vi "MFC_Setpoint.vi"(8 "error in":errorcluster, 9 "index":i32, 10 "MFC Set":T1[](array[typedef])=[{"MFC Set"=[{"String"="A", "MFC set"=1000.0}, {"String"="B", "MFC set"=100.0}], "set 1"=FALSE}] {"MFC Set"."MFC set" step=10.0 format="%.2f"}, 11 "VISA Refnum in":refnum<visa-resource-name>="COM6") -> (0 "error out":errorcluster, 3 "VISA Refnum out":refnum<visa-resource-name>="COM6")   [LabVIEW 2020]
uses:
  typeDefs/MFCSet.ctl
panel:
  out "MFC Index":i32
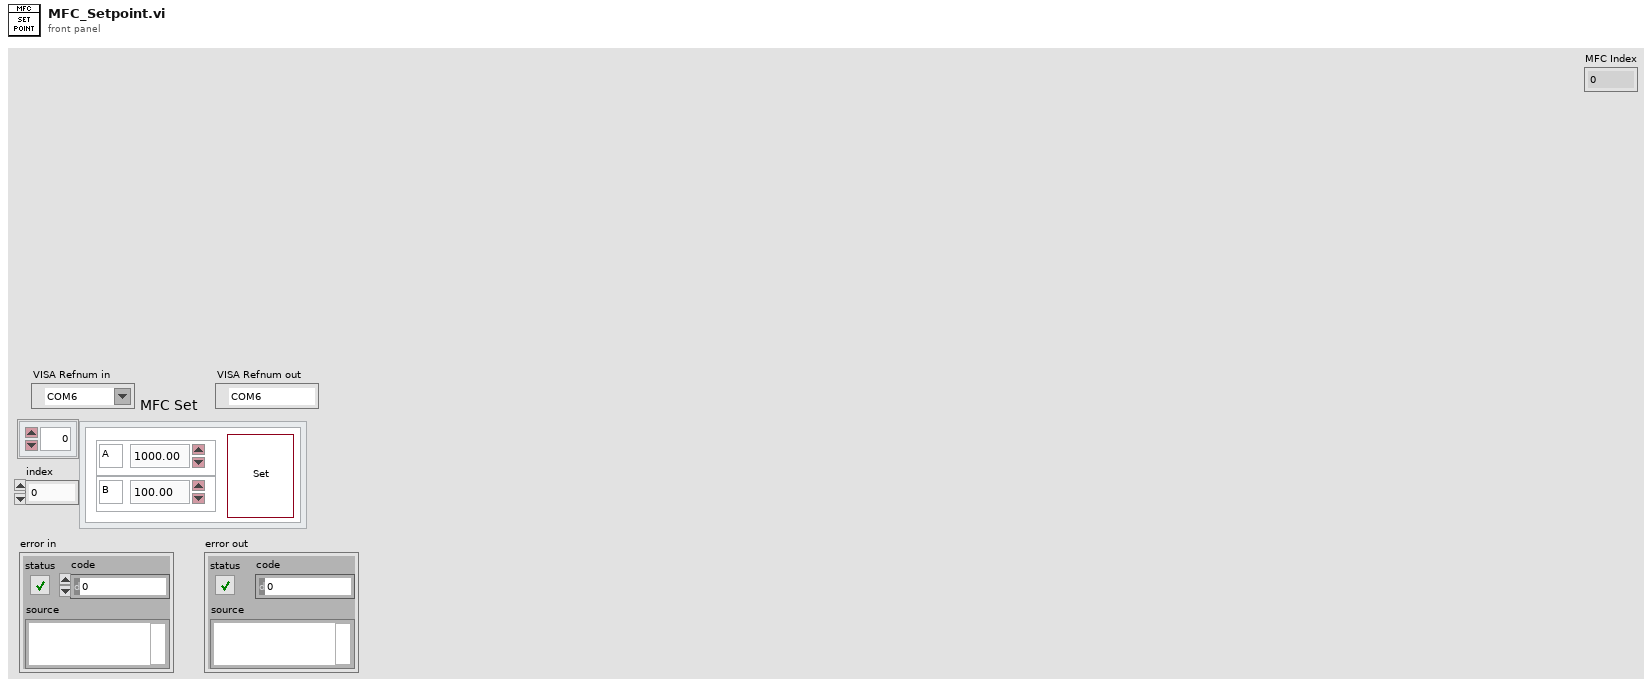
[diagram p1: front panel]
types:
  T1 = typedef "MFCSet.ctl" = cluster{"MFC Set":cluster{"String":string, "MFC set":dbl}[], "set 1":bool}
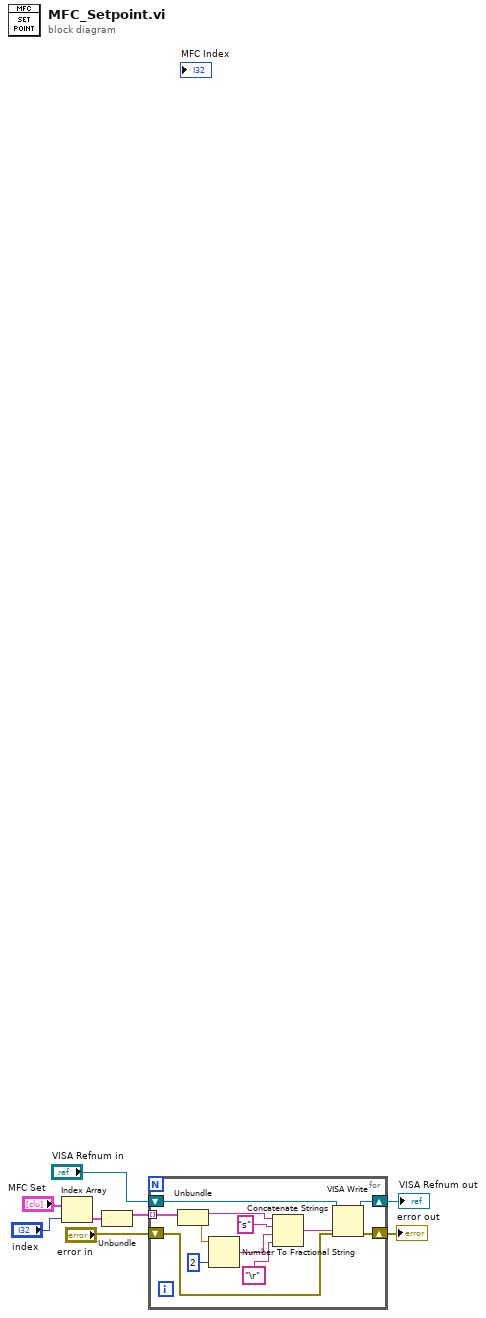
[diagram p0: block diagram]
diagram:
  n1 = Index Array(array="MFC Set", index="index") -> (element=w4:T1)
  n2 = Unbundle(w4) -> ("MFC Set"=w1:cluster{"String":string, "MFC set":dbl}[])  [unwired: 1 out]
  n3 = for {
    shift-right: [w9] -> w7
    shift-left: "error in" -> [w20]
    shift-right: [w10] -> w8
    shift-left: "VISA Refnum in" -> [w19]
    tunnel: w1 -> [w16] mode=indexing
    n4 = Unbundle(w16) -> ("String"=w15:string, "MFC set"=w14:dbl)
    n5 = Number To Fractional String(number=w14, precision (6)=i16 2) -> (F-format string=w12:string)  [unwired: 2 in]
    n6 = Concatenate Strings(w15, "s" ("string"), w12, "\r" ("string")) -> (w18:string)
    n7 = VISA Write(VISA resource name=w19, write buffer=w18, error in (no error)=w20) -> (VISA resource name out=w10:refnum<visa-resource-name>, error out=w9:errorcluster)  [unwired: 1 out]
  }
  "VISA Refnum out" <- w8
  "error out" <- w7
